vi "Read Server Internal UEs.vi"(8 "error in (no error)":errorcluster, 11 "ServiceName Template in":refnum<class "ServiceName Template.lvclass">) -> (0 "error out":errorcluster, 2 "Server Internal UEs":T1, 3 "ServiceName Template out":refnum<class "ServiceName Template.lvclass">)   [LabVIEW 2024, in "ServiceName Template.lvclass"]
uses:
  ServiceName Template.lvclass
  typeDefs/Server Internal UEs.ctl
  typeDefs/Server Internal Message.ctl
  ServiceName Template.lvclass/ServiceName Template.ctl
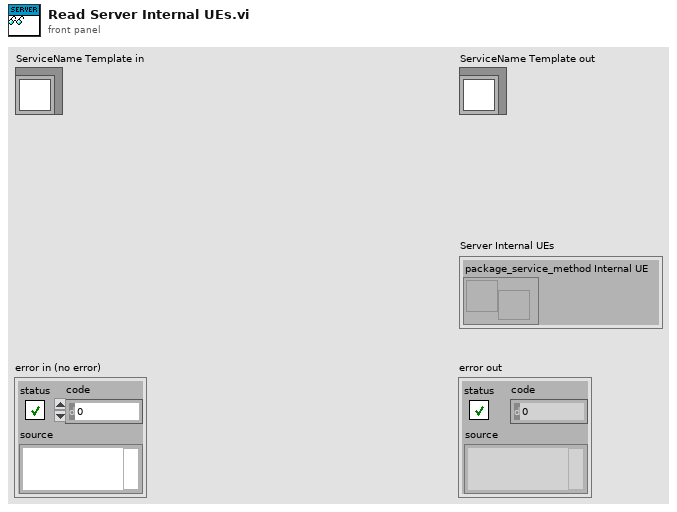
[diagram p1: front panel]
types:
  T1 = typedef "ServiceName Template.lvclass/Server Internal UEs.ctl" = cluster{"package_service_method Internal UE":refnum<user-event>}
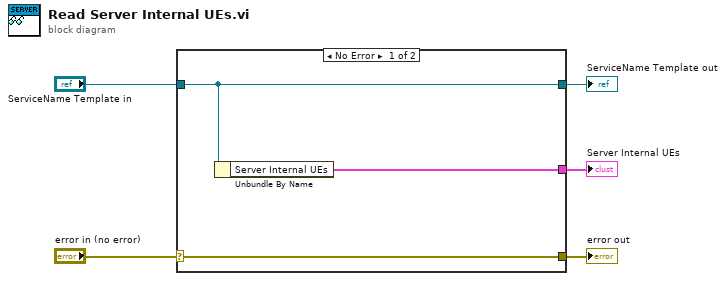
[diagram p0: block diagram]
diagram:
  n1 = case shown="No Error" "error in (no error)" {
    selector: "error in (no error)" -> [w8 w9]
    tunnel: [w8 w9] -> w4
    tunnel: [w7 w10] -> w2
    tunnel: "ServiceName Template in" -> [w7 w10]
    tunnel: [w6 _] -> w1
    frame No Error {
      n2 = Unbundle By Name(w7) -> ("Server Internal UEs"=w6:T1)
    }
    frame Error {
    }
  }
  "error out" <- w4
  "ServiceName Template out" <- w2
  "Server Internal UEs" <- w1
